vi "Exchange_Subtracks_Coordinates-1.vi"(5 "[IN] Subtrack wit\nhout prehistory":dbl[](array[numeric]), 6 "[IN] Row index \nProblem Point":i32, 7 "[IN] Subtrack \nwith problem":dbl[](array[numeric])) -> (1 "[OUT] Reconnected subtrack\n(posthistory after deleted \ncrossconnected point)":dbl[](array[numeric]), 3 "[OUT] Reconnected subtrack\nPrehistory + alternative prob\nlem point":dbl[](array[numeric]))   [LabVIEW 2013]
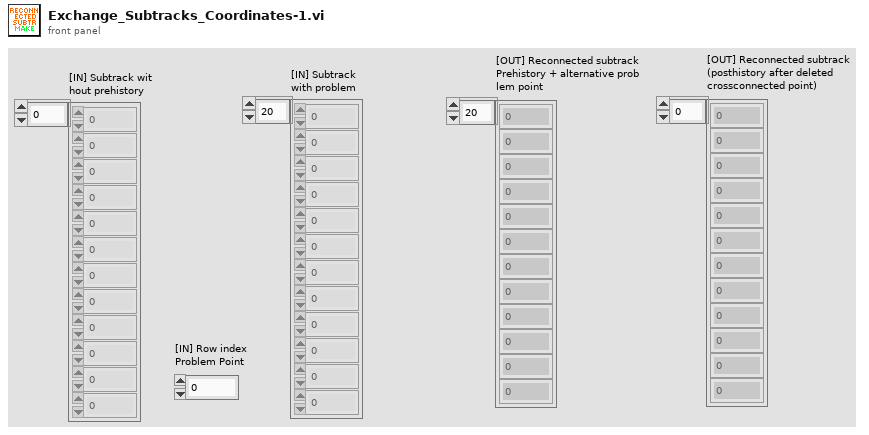
[diagram p1: front panel]
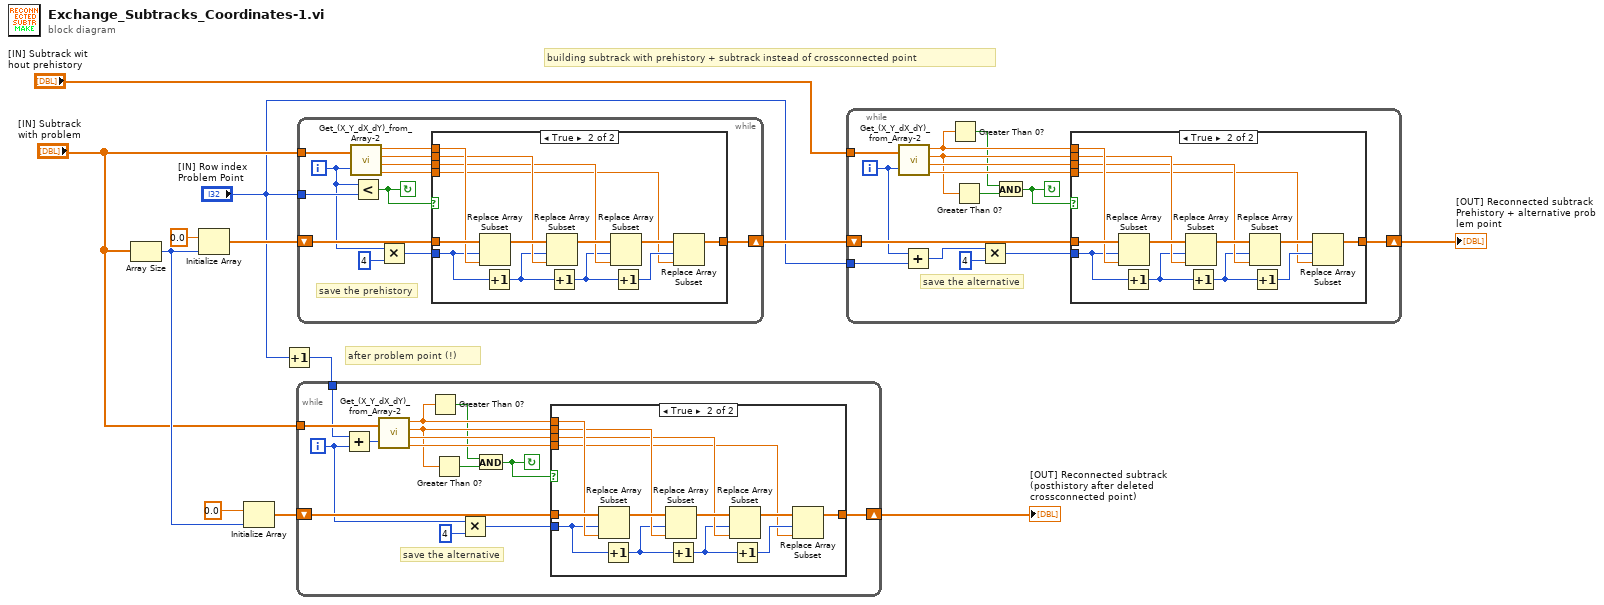
[diagram p0: block diagram]
diagram:
  # "after problem point (!)"
  # "building subtrack with prehistory + subtrack instead of crossconnected point"
  n1 = Array Size(array="[IN] Subtrack \nwith problem") -> (size(s)=w10:i32)
  n2 = Initialize Array(0.0 ("element"), w10) -> (w9:dbl[])
  n3 = Initialize Array(0.0 ("element"), w10) -> (w5:dbl[])
  n4 = Increment(x="[IN] Row index \nProblem Point") -> (x+1=w1:i32)
  n5 = while {
    shift-right: [w21] -> w3
    shift-left: w5 -> [w24]
    tunnel: "[IN] Subtrack \nwith problem" -> [w27]
    tunnel: w1 -> [w14]
    i -> [w15]
    stop <- w16 continue-if-true
    # "save the alternative"
    n6 = Add(x=w14, y=w15) -> (x+y=w13:i32)
    n7 = call "Get_(X_Y_dX_dY)_from_Array-2.vi"("(X,Y,dX,dY)"=w27, "Index of Displacement"=w13) -> ("X"=w20:dbl, "Y"=w19:dbl, "dX"=w26:dbl, "dY"=w25:dbl)
    n8 = Greater Than 0?(x=w20) -> (x > 0?=w17:bool)
    n9 = Greater Than 0?(x=w19) -> (x > 0?=w18:bool)
    n10 = Multiply(x=w15, y=4) -> (x*y=w22:i32)
    n11 = And(x=w17, y=w18) -> (x .and. y?=w16:bool)
    n12 = case shown="True" w16 {
      tunnel: w20 -> [_ w40]
      tunnel: w19 -> [_ w37]
      tunnel: w26 -> [_ w32]
      tunnel: w25 -> [_ w30]
      tunnel: w24 -> [w28 w41]
      tunnel: w22 -> [_ w39]
      tunnel: [w28 w29] -> w21
      frame False {
      }
      frame True {
        n13 = Replace Array Subset(array=w41, new element=w40, index=w39) -> (w38:dbl[])
        n14 = Increment(x=w39) -> (x+1=w36:i32)
        n15 = Replace Array Subset(array=w38, new element=w37, index=w36) -> (w33:dbl[])
        n16 = Increment(x=w36) -> (x+1=w31:i32)
        n17 = Replace Array Subset(array=w33, new element=w32, index=w31) -> (w35:dbl[])
        n18 = Increment(x=w31) -> (x+1=w34:i32)
        n19 = Replace Array Subset(array=w35, new element=w30, index=w34) -> (w29:dbl[])
      }
    }
  }
  "[OUT] Reconnected subtrack\n(posthistory after deleted \ncrossconnected point)" <- w3
  n20 = while {
    shift-right: [w42] -> w8
    shift-left: w9 -> [w46]
    tunnel: "[IN] Subtrack \nwith problem" -> [w53]
    tunnel: "[IN] Row index \nProblem Point" -> [w52]
    i -> [w45]
    stop <- w51 continue-if-true
    # "save the prehistory"
    n21 = call "Get_(X_Y_dX_dY)_from_Array-2.vi"("(X,Y,dX,dY)"=w53, "Index of Displacement"=w45) -> ("X"=w50:dbl, "Y"=w49:dbl, "dX"=w48:dbl, "dY"=w47:dbl)
    n22 = Less?(x=w45, y=w52) -> (x < y?=w51:bool)
    n23 = Multiply(x=w45, y=4) -> (x*y=w43:i32)
    n24 = case shown="True" w51 {
      tunnel: w50 -> [_ w66]
      tunnel: w49 -> [_ w63]
      tunnel: w48 -> [_ w58]
      tunnel: w47 -> [_ w56]
      tunnel: w46 -> [w54 w67]
      tunnel: w43 -> [_ w65]
      tunnel: [w54 w55] -> w42
      frame False {
      }
      frame True {
        n25 = Replace Array Subset(array=w67, new element=w66, index=w65) -> (w64:dbl[])
        n26 = Increment(x=w65) -> (x+1=w62:i32)
        n27 = Replace Array Subset(array=w64, new element=w63, index=w62) -> (w59:dbl[])
        n28 = Increment(x=w62) -> (x+1=w57:i32)
        n29 = Replace Array Subset(array=w59, new element=w58, index=w57) -> (w61:dbl[])
        n30 = Increment(x=w57) -> (x+1=w60:i32)
        n31 = Replace Array Subset(array=w61, new element=w56, index=w60) -> (w55:dbl[])
      }
    }
  }
  n32 = while {
    shift-right: [w76] -> w6
    shift-left: w8 -> [w79]
    tunnel: "[IN] Subtrack wit\nhout prehistory" -> [w82]
    tunnel: "[IN] Row index \nProblem Point" -> [w74]
    i -> [w75]
    stop <- w68 continue-if-true
    # "save the alternative"
    n33 = call "Get_(X_Y_dX_dY)_from_Array-2.vi"("(X,Y,dX,dY)"=w82, "Index of Displacement"=w75) -> ("X"=w72:dbl, "Y"=w71:dbl, "dX"=w81:dbl, "dY"=w80:dbl)
    n34 = Add(x=w75, y=w74) -> (x+y=w73:i32)
    n35 = Greater Than 0?(x=w72) -> (x > 0?=w69:bool)
    n36 = Greater Than 0?(x=w71) -> (x > 0?=w70:bool)
    n37 = Multiply(x=w73, y=4) -> (x*y=w77:i32)
    n38 = And(x=w69, y=w70) -> (x .and. y?=w68:bool)
    n39 = case shown="True" w68 {
      tunnel: w72 -> [_ w95]
      tunnel: w71 -> [_ w92]
      tunnel: w81 -> [_ w87]
      tunnel: w80 -> [_ w85]
      tunnel: w79 -> [w83 w96]
      tunnel: w77 -> [_ w94]
      tunnel: [w83 w84] -> w76
      frame False {
      }
      frame True {
        n40 = Replace Array Subset(array=w96, new element=w95, index=w94) -> (w93:dbl[])
        n41 = Increment(x=w94) -> (x+1=w91:i32)
        n42 = Replace Array Subset(array=w93, new element=w92, index=w91) -> (w88:dbl[])
        n43 = Increment(x=w91) -> (x+1=w86:i32)
        n44 = Replace Array Subset(array=w88, new element=w87, index=w86) -> (w90:dbl[])
        n45 = Increment(x=w86) -> (x+1=w89:i32)
        n46 = Replace Array Subset(array=w90, new element=w85, index=w89) -> (w84:dbl[])
      }
    }
  }
  "[OUT] Reconnected subtrack\nPrehistory + alternative prob\nlem point" <- w6
